vi "报警信息.vi"(8 "error in (no error)":errorcluster, 11 "data":T1) -> (0 "error out":errorcluster)   [LabVIEW 2016, in "数据传输系统-05.lvlib"]
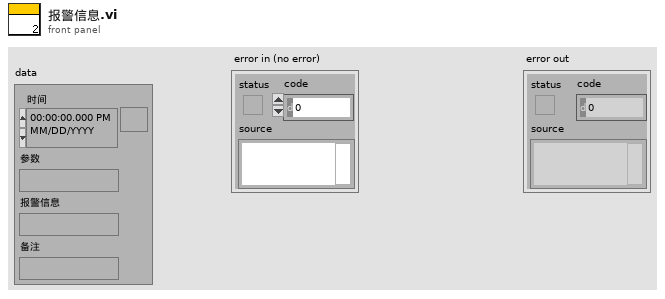
[diagram p1: front panel]
types:
  T1 = typedef "报警信息字段定义.ctl" = cluster{"时间":timestamp, "参数":string, "报警信息":string, "备注":string}
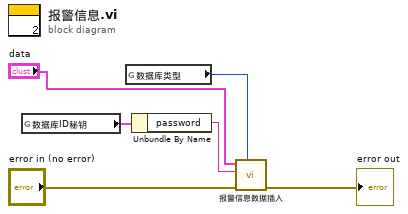
[diagram p0: block diagram]
diagram:
  n1 = global read "外部交互全局.vi" "数据库ID秘钥"() -> (w2:cluster{"userID":string, "password":string})
  n2 = global read "断电保存全局.vi" "数据库类型"() -> (w6:enum16{"Access", "SQLite"})
  n3 = Unbundle By Name(w2) -> ("password"=w1:string)
  n4 = call "报警信息数据插入.vi"("data"="data", "Password"=w1, "错误输入（无错误）"="error in (no error)", "数据库类型"=w6) -> ("错误输出"=→"error out":errorcluster)  [unwired: 6 in]
